vi "SDSU_Memory.vi"(0 "refnum":i32, 1 "Database RefNum in":T1, 5 "Command In":string, 7 "physical unit":string, 11 "error in (no error)":errorcluster) -> (4 "refnum out":i32, 6 "message":string, 8 "Read Value":i32, 15 "error out":errorcluster)   [LabVIEW 2016]
doc: "This VI passes the addressing information in the instrument decriptor to the Instr Open VI and returns the instrument ID. You can optionally reset the instrument by setting the front panel reset control. You must run this VI before using any of the instrument driver VIs for this instrument."
uses:
  DBSHAND/private/vis/DatabaseHand_RefNum.ctl
  DBSHAND/private/vis/DatabaseHand_Element_Set(string).vi
  SDSU_GBLVariables.vi
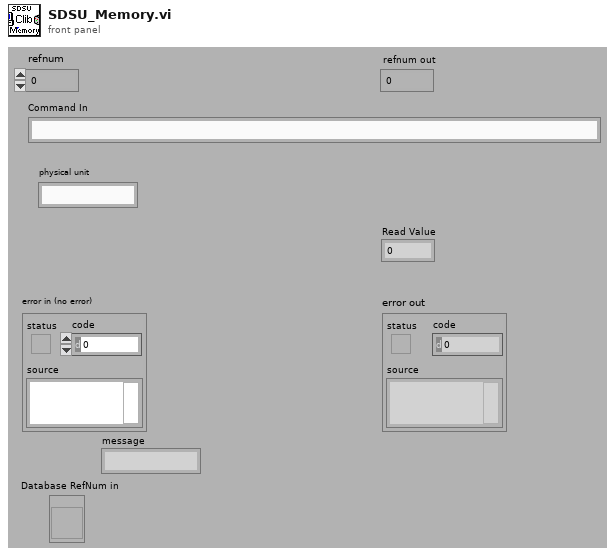
[diagram p1: front panel]
types:
  T1 = typedef "DatabaseHand_RefNum.ctl" = refnum<vi>
  T2 = enum16{"set all", "set", "get all", "get list", "get"}
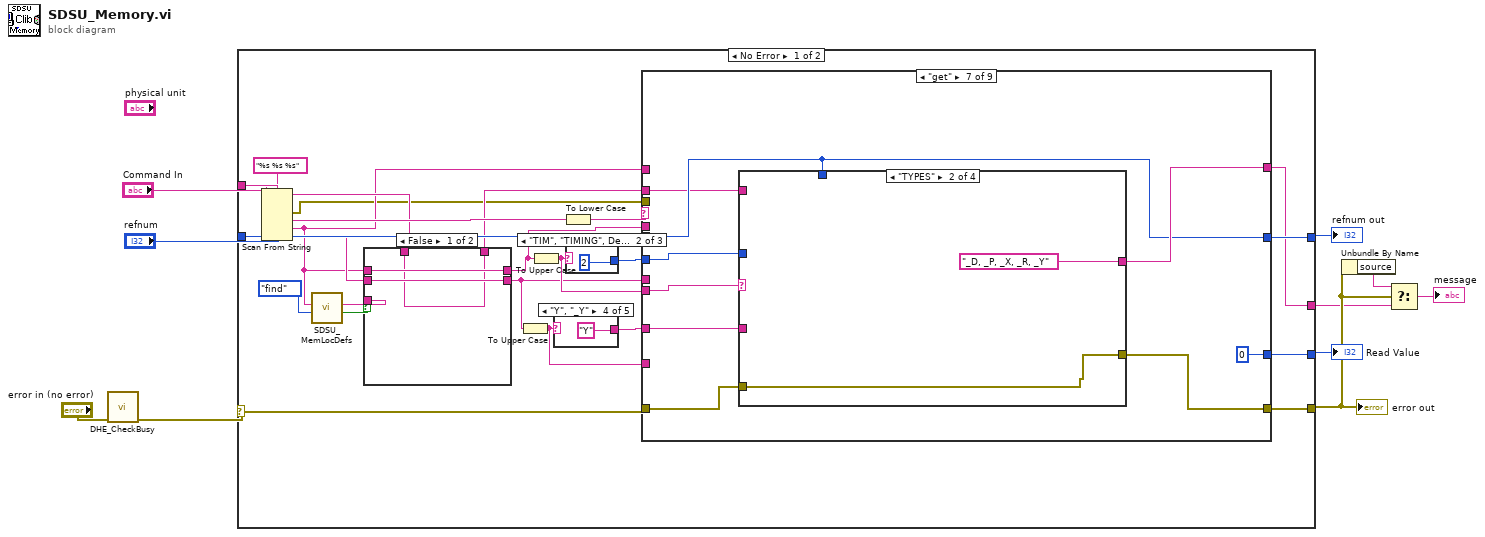
[diagram p0: block diagram]
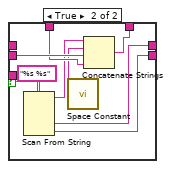
[diagram p2: hidden frame]
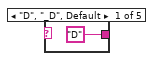
[diagram p3: hidden frame]
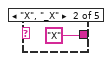
[diagram p4: hidden frame]
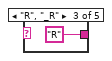
[diagram p5: hidden frame]
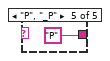
[diagram p6: hidden frame]
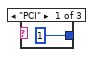
[diagram p7: hidden frame]
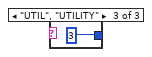
[diagram p8: hidden frame]
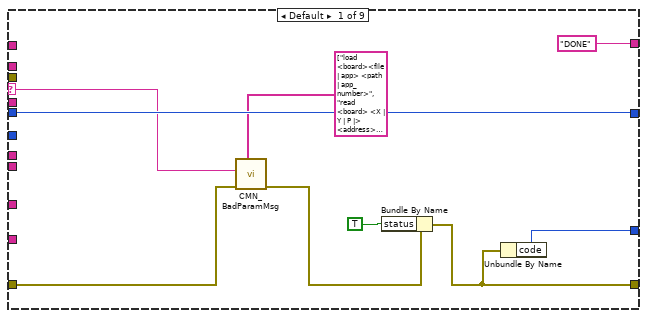
[diagram p9: hidden frame]
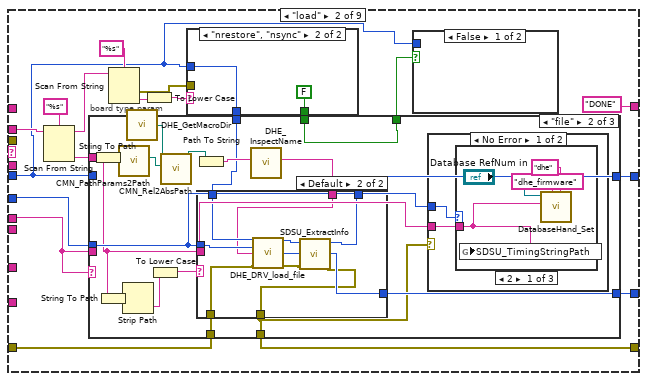
[diagram p10: hidden frame]
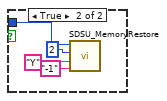
[diagram p11: hidden frame]
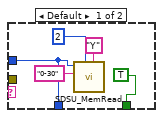
[diagram p12: hidden frame]
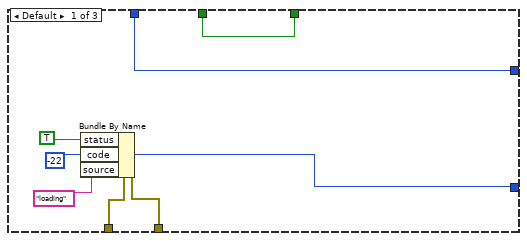
[diagram p13: hidden frame]
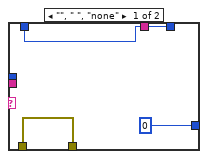
[diagram p14: hidden frame]
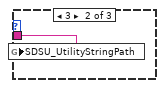
[diagram p15: hidden frame]
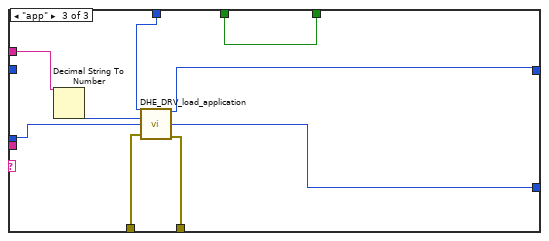
[diagram p18: hidden frame]
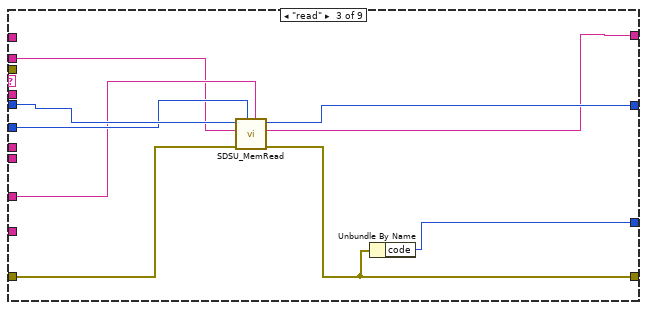
[diagram p19: hidden frame]
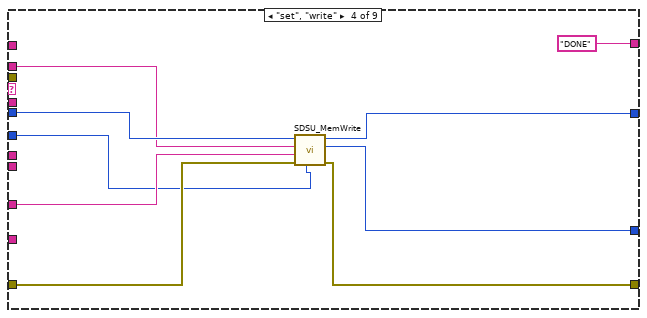
[diagram p20: hidden frame]
diagram:
  n1 = call "DHE_CheckBusy.vi"("error in (no error)"="error in (no error)") -> ("error out"=w1:errorcluster)  [unwired: 2 in, 8 out]
  n2 = case shown="No Error" w1 {
    selector: w1 -> [w30 w273]
    tunnel: [w34 w273] -> w5
    tunnel: "refnum" -> [w33 w274]
    tunnel: [w32 w274] -> w9
    tunnel: "Command In" -> [w29 _]
    tunnel: [w31 w272] -> w7
    tunnel: [w23 "ERR" ("f")] -> w2
    frame No Error {
      n3 = Scan From String(format string="%s %s %s" ("Format String"), input string=w29) -> (remaining string=w14:string, error out=w11:errorcluster, output 1=w27:string, output 2=w12:string, output 3=w17:string)  [unwired: 2 in, 4 out]
      n4 = call "SDSU_MemLocDefs.vi"("action"=enum16{"read from file", "find", "clear"}."find", "name"=w12) -> ("found"=w19:bool, "location"=w15:string)  [unwired: 7 in, 1 out]
      n5 = case shown="False" w19 {
        tunnel: w12 -> [w37 _]
        tunnel: [w37 w44] -> w18
        tunnel: w17 -> [w36 w42]
        tunnel: [w36 w43] -> w16
        tunnel: w15 -> [_ w45]
        tunnel: w14 -> [w35 w41]
        tunnel: [w35 w40] -> w13
        frame False {
        }
        frame True {
          n6 = Scan From String(format string="%s %s", input string=w45) -> (remaining string=w39:string, output 1=w44:string, output 2=w43:string)  [unwired: 4 in, 2 out]
          n7 = call <vilib>:"Space Constant.vi"() -> ("String"=w38:string)
          n8 = Concatenate Strings(w39, w38, w42, w41) -> (w40:string)
        }
      }
      n9 = To Upper Case(1:w16) -> (0:w21:string)
      n10 = To Upper Case(1:w18) -> (0:w22:string)
      n11 = case shown="\"Y\", \"_Y\"" w21 {
        tunnel: ["D" "X" "R" "Y" "P"] -> w26
        frame "D", "_D", Default {
        }
        frame "X", "_X" {
        }
        frame "R", "_R" {
        }
        frame "Y", "_Y" {
        }
        frame "P", "_P" {
        }
      }
      n12 = To Lower Case(string=w27) -> (all lower case string=w24:string)
      n13 = case shown="\"TIM\", \"TIMING\", Default" w22 {
        tunnel: [i16 1 i16 2 i16 3] -> w25
        frame "PCI" {
        }
        frame "TIM", "TIMING", Default {
        }
        frame "UTIL", "UTILITY" {
        }
      }
      n14 = case shown="\"get\"" w24 {
        selector: w24 -> [w61 _ _ _ _ _ _ _ _]
        tunnel: w30 -> [w62 w81 w151 w161 w175 _ w187 w235 w248]
        tunnel: [w57 w80 w147 w160 w172 w177 w186 w234 w248] -> w34
        tunnel: w33 -> [w63 w66 w154 w162 w173 w182 w190 w237 w242]
        tunnel: [w63 w82 w153 w159 w173 w181 w190 w236 w242] -> w32
        tunnel: w26 -> [_ _ w149 w156 _ w179 w189 _ _]
        tunnel: [w60 w79 w146 w158 w171 w185 0 ("error_code") w233 0 ("error_code")] -> w31
        tunnel: w16 -> [_ w77 _ _ w169 _ _ w231 w241]
        tunnel: w25 -> [_ w78 w150 w155 w170 w180 w191 w232 _]
        tunnel: w13 -> [_ w76 w148 w157 _ w176 w188 w239 w240]
        tunnel: ["DONE" ("f") "DONE" ("f") w152 "DONE" ("f") w174 "DONE" ("response") w193 "DONE" ("f") w245] -> w23
        tunnel: w22 -> [_ _ _ _ _ _ w194 _ w247]
        tunnel: w21 -> [_ _ _ _ _ _ _ _ w244]
        tunnel: w18 -> [_ _ _ _ _ _ _ _ w243]
        tunnel: w12 -> [_ _ _ _ _ w184 _ _ _]
        tunnel: w11 -> [_ _ _ _ _ _ _ _ _]
        frame Default {
          n15 = call "CMN_BadParamMsg.vi"("valid params"=string[] ["load  <board><file  | app> <path | app_number>", "read  <board> <X | Y | P |> <address>", "write <board> <X | Y | P> <address> <value>", "manualcommand <tim | util | pci> <arg1 | none> <arg2 | none> ...<arg5 | none> <command>"], "error in (no error)"=w62, "parameter"=w61) -> ("error out"=w58:errorcluster)  [unwired: 1 in, 7 out]
          n16 = Bundle By Name(cluster=w58, "status"=TRUE) -> (w57:errorcluster)
          n17 = Unbundle By Name(w57) -> ("code"=w60:i32)
        }
        frame "load" {
          # "board type param"
          n18 = Scan From String(format string="%s" ("Format String"), input string=w76) -> (remaining string=w72:string, output 1=w74:string)  [unwired: 2 in, 3 out]
          n19 = Scan From String(format string="%s", input string=w72) -> (error out=w65:errorcluster, output 1=w70:string)  [unwired: 2 in, 3 out]
          n20 = To Lower Case(string=w70) -> (all lower case string=w64:string)
          n21 = case shown="\"nrestore\", \"nsync\"" w64 {
            tunnel: w66 -> [w91 w93]
            tunnel: [w91 w93] -> w69
            tunnel: [TRUE FALSE] -> w68
            tunnel: w65 -> [_ _]
            frame Default {
              n22 = call "SDSU_MemRead.vi"("type"="Y", "board dest"=i16 2, "memin"="0-30", "fd"=w91) -> ()  [unwired: 1 in, 7 out]
            }
            frame "nrestore", "nsync" {
            }
          }
          n23 = case shown="\"file\"" w77 {
            tunnel: w66 -> [_ _ _]
            tunnel: [w95 w115 w143] -> w82
            tunnel: w81 -> [w100 w117 w145]
            tunnel: [w99 w112 w144] -> w80
            tunnel: [w96 w116 w139] -> w79
            tunnel: w78 -> [_ w114 w140]
            tunnel: w77 -> [_ _ _]
            tunnel: w74 -> [_ w105 w142]
            tunnel: w69 -> [w95 w102 w138]
            tunnel: w68 -> [w94 w101 w137]
            tunnel: [w94 w101 w137] -> w67
            frame Default {
              w96 = -22
              n24 = Bundle By Name(cluster=w100, "status"=TRUE, "code"=w96, "source"="loading") -> (w99:errorcluster)
            }
            frame "file" {
              n25 = String To Path(string=w105) -> (path=w107:path)
              n26 = String To Path(string=w105) -> (path=w104:path)
              n27 = call "CMN_PathParams2Path.vi"("Path In"=w107) -> ("Path out"=w108:path)  [unwired: 2 in, 8 out]
              n28 = Strip Path(path=w104) -> (name=w103:string)  [unwired: 1 out]
              n29 = call "DHE_GetMacroDir.vi"() -> ("DHE_MacroDir"=w109:path)  [unwired: 9 out]
              n30 = To Lower Case(string=w103) -> (all lower case string=w113:string)
              n31 = call "CMN_Rel2AbsPath.vi"("test path"=w108, "absolute path"=w109) -> ("output path"=w110:path)  [unwired: 1 in, 8 out]
              n32 = Path To String(path=w110) -> (string=w111:string)
              n33 = call "DHE_InspectName.vi"("name in"=w111) -> ("name out"=w106:string)  [unwired: 10 out]
              n34 = case shown="Default" w113 {
                tunnel: w102 -> [w119 w129]
                tunnel: w117 -> [w120 w128]
                tunnel: [0 ("return value") w127] -> w116
                tunnel: [w119 w124] -> w115
                tunnel: w114 -> [_ w123]
                tunnel: w105 -> [_ _]
                tunnel: [w120 w122] -> w112
                tunnel: w106 -> [_ w121]
                frame "", " ", "none" {
                }
                frame Default {
                  n35 = call "DHE_DRV_load_file.vi"("fd"=w129, "dest"=w123, "filename"=w121, "error in (no error)"=w128) -> ("fd out"=w126:i32, "return value"=w127:i32, "error out"=w125:errorcluster)  [unwired: 9 out]
                  n36 = call "SDSU_ExtractInfo.vi"("error in (no error)"=w125, "refnum"=w126) -> ("error out"=w122:errorcluster, "refnum out"=w124:i32)  [unwired: 8 out]
                }
              }
              n37 = case shown="No Error" w112 {
                tunnel: w114 -> [w131 _]
                tunnel: w105 -> [w130 _]
                frame No Error {
                  n38 = case shown="2" w131 {
                    tunnel: w130 -> [w132 w136 _]
                    frame 2 {
                      n39 = global write "SDSU_GBLVariables.vi" "SDSU_TimingStringPath"(w132) -> ()
                      n40 = call-poly "DatabaseHand_Set.vi"("group"="dhe", "name"="dhe_firmware", "value"=w132, "Database RefNum in"="Database RefNum in") -> ()  [unwired: 4 in, 4 out]
                    }
                    frame 3 {
                      n41 = global write "SDSU_GBLVariables.vi" "SDSU_UtilityStringPath"(w136) -> ()
                    }
                    frame 1, Default {
                    }
                  }
                }
                frame Error {
                }
              }
            }
            frame "app" {
              n42 = Decimal String To Number(string=w142) -> (number=w141:i32)  [unwired: 3 out]
              n43 = call "DHE_DRV_load_application.vi"("fd"=w138, "app"=w141, "dest"=w140, "error in (no error)"=w145) -> ("fd out"=w143:i32, "return value"=w139:i32, "error out"=w144:errorcluster)  [unwired: 9 out]
            }
          }
          n44 = case shown="False" w67 {
            tunnel: w66 -> [_ w86]
            frame False {
            }
            frame True {
              n45 = call "SDSU_MemoryRestore.vi"("address"="-1", "type"="Y", "board"=i16 2, "refnum"=w86) -> ()  [unwired: 6 in, 2 out]
            }
          }
        }
        frame "read" {
          n46 = call "SDSU_MemRead.vi"("type"=w149, "board dest"=w150, "error in (no error)"=w151, "memin"=w148, "fd"=w154) -> ("error out"=w147:errorcluster, "values"=w152:string, "fd out"=w153:i32)  [unwired: 4 out]
          n47 = Unbundle By Name(w147) -> ("code"=w146:i32)
        }
        frame "set", "write" {
          n48 = call "SDSU_MemWrite.vi"("board dest"=w155, "error in (no error)"=w161, "type"=w156, "args"=w157, "fd"=w162) -> ("error out"=w160:errorcluster, "return value"=w158:i32, "fd out"=w159:i32)  [unwired: 4 out]
        }
        frame "dump" {
          n49 = Scan From String(format string="%d", input string=w169) -> (error out=w167:errorcluster, output 1=w166:i32)  [unwired: 2 in, 3 out]
          n50 = Select(t=31, s=w167, f=w166) -> (s? t:f=w165:i32)
          n51 = call "SDSU_MemDump.vi"("maxloc"=w165, "error in (no error)"=w175, "board dest"=w170, "refnum"=w173) -> ("error out"=w172:errorcluster, "mem"=w174:string)  [unwired: 1 in, 5 out]
          n52 = Unbundle By Name(w172) -> ("code"=w171:i32)
        }
        frame "restore" {
          n53 = To Lower Case(string=w184) -> (all lower case string=w178:string)
          n54 = call "SDSU_MemoryRestore.vi"("arg"=w178, "address"=w176, "type"=w179, "board"=w180, "refnum"=w182) -> ("error out"=w177:errorcluster, "refnum out"=w181:i32)  [unwired: 5 in]
          n55 = Unbundle By Name(w177) -> ("code"=w185:i32)
        }
        frame "get" {
          n56 = case shown="\"TYPES\"" w194 {
            selector: w194 -> [_ _ _ w217]
            tunnel: [w199 "_D, _P, _X, _R, _Y" w211 w212] -> w193
            tunnel: w191 -> [_ _ w210 _]
            tunnel: w190 -> [_ _ w209 _]
            tunnel: w189 -> [_ _ w208 _]
            tunnel: w188 -> [_ _ w207 _]
            tunnel: w187 -> [w195 w203 w205 w216]
            tunnel: [w195 w203 w206 w215] -> w186
            frame "BOARDS", "CARDS" {
              w196 = "\n"
              n57 = Concatenate Strings("name= PCI, address= 1 ", w196, "name= TIM, address= 2 ", w196, "name= UTIL, address= 3 ", w196, "name= VID, address= 4 ", w196, "name= CLK, address= 5") -> (w199:string)
            }
            frame "TYPES" {
            }
            frame "PCI", "TIM", "TIMING", "UTIL", "UTILITY" {
              n58 = call "SDSU_MemRead.vi"("type"=w208, "board dest"=w210, "error in (no error)"=w205, "memin"=w207, "fd"=w209) -> ("error out"=w206:errorcluster, "values"=w211:string)  [unwired: 5 out]
            }
            frame Default {
              n59 = Concatenate Strings("ERROR unknown memory location " ("string"), w217) -> (w212:string)
              n60 = Bundle By Name(cluster=w216, "status"=TRUE, "code"=-22, "source"=w212) -> (w215:errorcluster)
            }
          }
        }
        frame "manualcommand" {
          w226 = "none" ("search string")
          # "dest arg1 arg2 arg3 arg4 arg5 comm"
          n61 = Scan From String(format string="%s %s %s %s %s" ("Format String"), input string=w239) -> (output 1=w230:string, output 2=w229:string, output 3=w228:string, output 4=w227:string, output 5=w220:string)  [unwired: 2 in, 8 out]
          n62 = Search and Replace String(input string=w230, search string=w226) -> (result string=w224:string)  [unwired: 1 in, 8 out]
          n63 = Search and Replace String(input string=w231, search string=w226) -> (result string=w225:string)  [unwired: 1 in, 8 out]
          n64 = Search and Replace String(input string=w229, search string=w226) -> (result string=w223:string)  [unwired: 1 in, 8 out]
          n65 = Search and Replace String(input string=w228, search string=w226) -> (result string=w222:string)  [unwired: 1 in, 8 out]
          n66 = Search and Replace String(input string=w227, search string=w226) -> (result string=w221:string)  [unwired: 1 in, 8 out]
          n67 = call "DHE_DRV_manual_command.vi"("arg3"=w223, "arg4"=w222, "arg5"=w221, "command"=w220, "short board_dest"=w232, "error in (no error)"=w235, "arg2"=w224, "arg1"=w225, "fd"=w237) -> ("fd"=w236:i32, "error_code"=w233:i32, "error out"=w234:errorcluster)  [unwired: 8 out]
        }
        frame "clk", "clock", "mux" {
          n68 = case shown="\"GET\"" w247 {
            tunnel: ["ERROR unknow command to mux" ("f") w253 w257 w269] -> w245
            tunnel: w244 -> [_ _ w258 w268]
            tunnel: w243 -> [_ _ w256 _]
            tunnel: w242 -> [_ w255 _ _]
            tunnel: w241 -> [_ w252 _ _]
            tunnel: w240 -> [_ w251 _ w267]
            frame Default {
            }
            frame "SET" {
              n69 = Concatenate Strings(w252, w251) -> (w250:string)
              n70 = call "SDSU_ReadMux.vi"("fd"=w255, "argument"=w250, "action"=T2."set") -> ("response"=w253:string)  [unwired: 2 in, 6 out]
            }
            frame "GET" {
              n71 = case shown="Default" w258 {
                selector: w258 -> [w259 _ _]
                tunnel: [w260 w262 w264] -> w257
                tunnel: w256 -> [_ _ _]
                frame Default {
                  n72 = call "SDSU_ReadMux.vi"("argument"=w259, "action"=T2."get") -> ("response"=w260:string)  [unwired: 3 in, 6 out]
                }
                frame "LIST", "MUXLIST" {
                  n73 = call "SDSU_ReadMux.vi"("action"=T2."get list") -> ("response"=w262:string)  [unwired: 4 in, 6 out]
                }
                frame "CLKLIST", "CLKS" {
                  n74 = call "SDSU_ReadMux.vi"("action"=T2."get all") -> ("response"=w264:string)  [unwired: 4 in, 6 out]
                }
              }
            }
            frame "GETALL" {
              n75 = Concatenate Strings(w268, w267) -> (w266:string)
              n76 = call "SDSU_ReadMux.vi"("argument"=w266, "action"=T2."get all") -> ("response"=w269:string)  [unwired: 3 in, 6 out]
            }
          }
        }
      }
    }
    frame Error {
      n77 = Unbundle By Name(w273) -> ("code"=w272:i32)
    }
  }
  "error out" <- w5
  "refnum out" <- w9
  "Read Value" <- w7
  n78 = Unbundle By Name(w5) -> ("source"=w4:string)
  n79 = Select(t=w4, s=w5, f=w2) -> (s? t:f=→"message":string)
